vi "rethinkdb_handshake_client_final.vi"(8 "error in (no error)":errorcluster, 9 "client_first_message":string, 10 "password":string, 11 "server_response (json)":string="{\"success\":true,\"min_protocol_version\":0,\"max_protocol_version\":0,\"server_version\":\"2.3.0\"}\u0000\n{\"success\":true,\"authentication\":\"r=rOprNGfwEbeRWgbNEkqO%hvYDpWUa2RaTCAfuxFIlj)hNlF$k0,s=W22ZaJ0SNY7soEsUEjb6gQ==,i=4096\"}\u0000") -> (0 "error out":errorcluster, 3 "authentication_request":string)   [LabVIEW 2017]
uses:
  b02b9132-5309-4610-a6c0-a0c94150cd68.vi
  dab8a8d9-9bd0-4e10-b8f7-9264eab402ee.vi
  json/json_resolve_key.vi
panel:
  out "success?":bool
  out "server_first_message":string
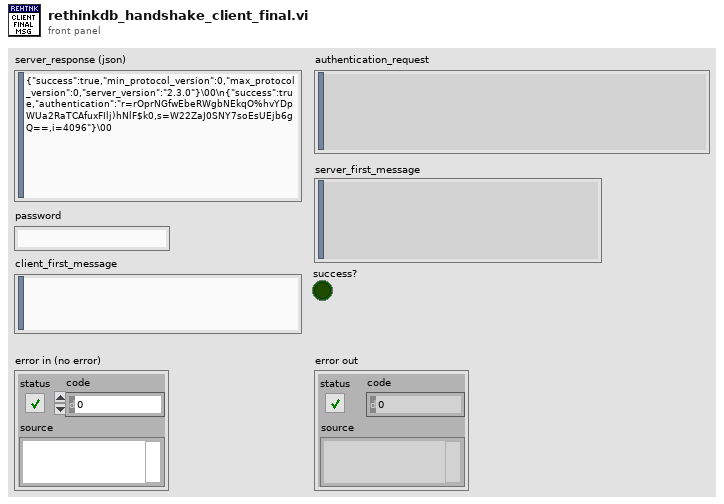
[diagram p1: front panel]
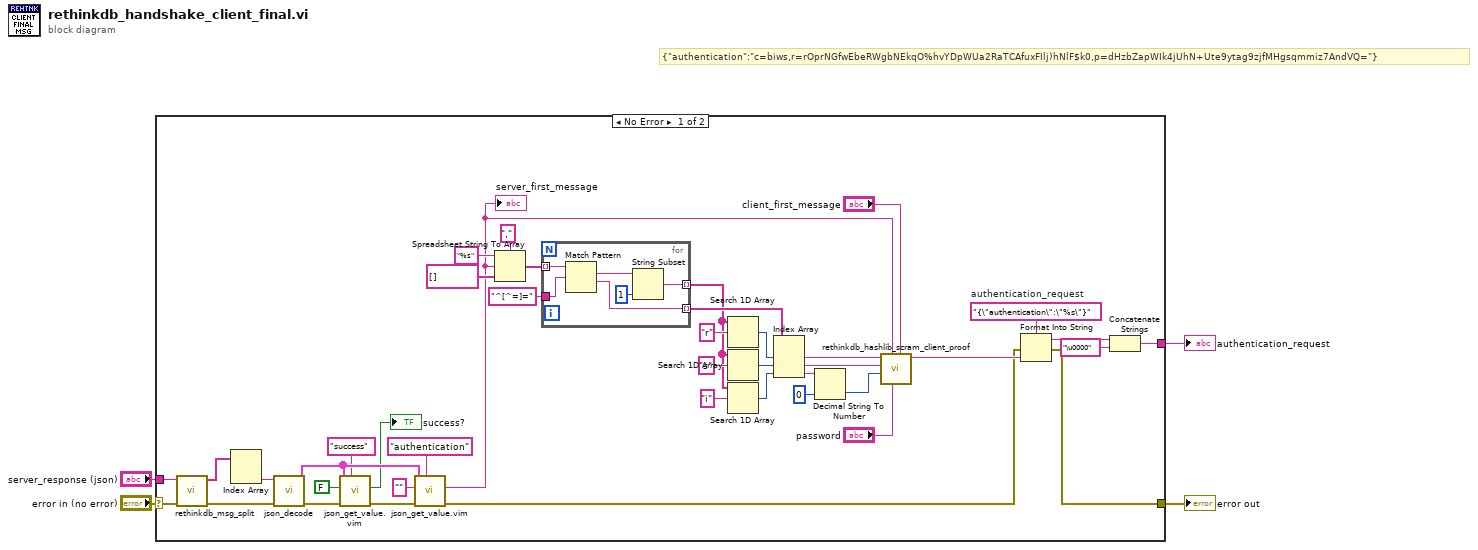
[diagram p0: block diagram]
diagram:
  # "{\"authentication\":\"c=biws,r=rOprNGfwEbeRWgbNEkqO%hvYDpWUa2RaTCAfuxFIlj)hNlF$k0,p=dHzbZapWIk4jUhN+Ute9ytag9zjfMHgsqmmiz7AndVQ=\"}"
  n1 = case shown="No Error" "error in (no error)" {
    selector: "error in (no error)" -> [w45 w52]
    tunnel: [w43 w52] -> w3
    tunnel: [w42 _] -> w2
    tunnel: "server_response (json)" -> [w44 _]
    frame No Error {
      w37 = "{\"authentication\":\"%s\"}"  # authentication_request
      n2 = call "rethinkdb_msg_split.vi"("error in (no error)"=w45, "data in"=w44) -> ("error out"=w29:errorcluster, "messages"=w38:string[])  [unwired: 7 in, 1 out]
      n3 = Index Array(array=w38) -> (element #2=w34:string)  [unwired: 2 in, 1 out]
      n4 = call "json_decode.vi"("error in (no error)"=w29, "json"=w34) -> ("error out"=w33:errorcluster, "pairs"=w31:cluster{"key":string, "value":variant}[])  [unwired: 8 in]
      n5 = call "json_get_value.vim"("key"="success", "error in (no error)"=w33, "default"=FALSE, "pairs"=w31) -> ("error out"=w32:errorcluster, "value"=→"success?":bool)  [unwired: 5 in, 1 out]
      n6 = call "json_get_value.vim"("key"="authentication", "error in (no error)"=w32, "default"="", "pairs"=w31) -> ("error out"=w10:errorcluster, "value"=w5:string)  [unwired: 5 in, 1 out]
      "server_first_message" <- w5
      n7 = Spreadsheet String To Array(delimiter (Tab)=",", format string="%s", spreadsheet string=w5, array type (2D Dbl)=string[] []) -> (array=w24:string[])
      n8 = for {
        tunnel: w24 -> [w51] mode=indexing
        tunnel: [w47] -> w16 mode=indexing
        tunnel: [w50] -> w21 mode=indexing
        tunnel: "^[^=]=" ("regular expression") -> [w49]
        n9 = Match Pattern(string=w51, regular expression=w49) -> (match substring=w46:string, after substring=w50:string)  [unwired: 1 in, 2 out]
        n10 = String Subset(string=w46, length (rest)=1 ("length (rest)")) -> (substring=w47:string)  [unwired: 1 in]
      }
      n11 = Search 1D Array(1D array=w16, element="r") -> (index of element=w19:i32)  [unwired: 1 in]
      n12 = Search 1D Array(1D array=w16, element="s") -> (index of element=w18:i32)  [unwired: 1 in]
      n13 = Search 1D Array(1D array=w16, element="i") -> (index of element=w15:i32)  [unwired: 1 in]
      n14 = Index Array(array=w21, index #1=w19, index #2=w18, index #3=w15) -> (element #1=w12:string, element #2=w13:string, element #3=w14:string)
      n15 = Decimal String To Number(string=w14, default (0L)=0 ("default (0 I32)")) -> (number=w9:i32)  [unwired: 1 in, 1 out]
      n16 = call "rethinkdb_hashlib_scram_client_proof.vi"("client_first_message"="client_first_message", "password"="password", "server_first_message"=w5, "i"=w9, "s"=w13, "r"=w12) -> ("client_final_msg"=w11:string)  [unwired: 5 in]
      n17 = Format Into String(format string=w37, error in=w10, w11) -> (resulting string=w36:string, error out=w43:errorcluster)  [unwired: 1 in]
      n18 = Concatenate Strings(w36, "\u0000" ("string")) -> (w42:string)
    }
    frame Error {
    }
  }
  "error out" <- w3
  "authentication_request" <- w2
